vi "Play System Sound.vi"(8 "Error In":errorcluster, 11 "Windows Sound":T1) -> (0 "Error Out":errorcluster)   [LabVIEW 2021, in "Sound.lvlib"]
uses:
  Sound.lvlib
  System Sounds List.ctl
  <vilib>/Utility/sysdir.llb/System Directory Type.ctl
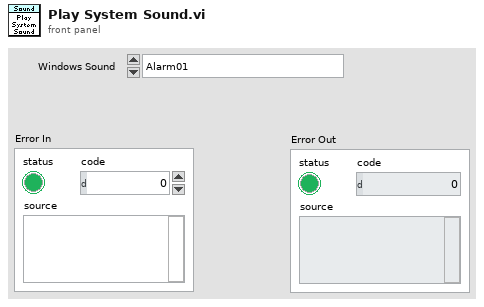
[diagram p1: front panel]
types:
  T1 = typedef "Sound.lvlib/System Sounds List.ctl" = enum16{"Alarm01", "Alarm02", "Alarm03", "Alarm04", "Alarm05", "Alarm06", "Alarm07", "Alarm08", "Alarm09", "Alarm10", "chimes", "chord", "ding", "notify", "recycle", "Ring01", "Ring02", "Ring03", "Ring04", "Ring05", "Ring06", "Ring07", "Ring08", "Ring09", "Ring10", "ringout", "Speech Off", "Speech On", "Speech Sleep", "tada", "Windows Background", "Windows Balloon", "Windows Battery Critical", "Windows Battery Low", "Windows Critical Stop", "Windows Default", "Windows Ding", "Windows Error", "Windows Exclamation", "Windows Feed Discovered", "Windows Foreground", "Windows Hardware Fail", "Windows Hardware Insert", "Windows Hardware Remove", "Windows Information Bar", "Windows Logoff Sound", "Windows Logon", "Windows Menu Command", "Windows Message Nudge", "Windows Minimize", "Windows Navigation Start", "Windows Notify Calendar", "Windows Notify Email", "Windows Notify Messaging", "Windows Notify System Generic", "Windows Notify", "Windows Pop-up Blocked", "Windows Print complete", "Windows Proximity Connection", "Windows Proximity Notification", "Windows Recycle", "Windows Restore", "Windows Ringin", "Windows Ringout", "Windows Shutdown", "Windows Startup", "Windows Unlock", "Windows User Account Control"}
  T2 = typedef "System Directory Type.ctl" = i32
  T3 = typedef "Sound Output Task ID.ctl" = u32
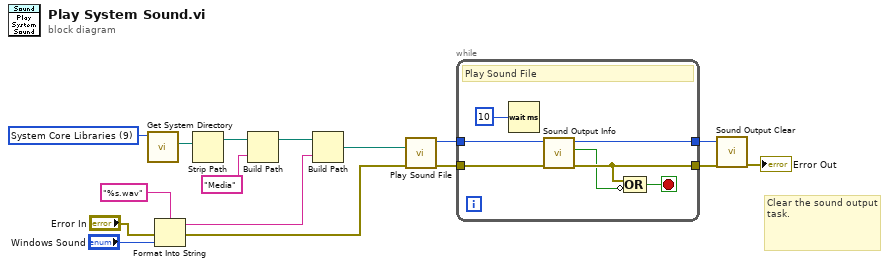
[diagram p0: block diagram]
diagram:
  w14 = T2 9 items=["User Home"=0, "User Desktop"=1, "User Documents"=2, "User Application Data"=3, "User Preferences"=4, "User Temporary"=5, "Public Documents"=6, "Public Application Data"=7, "Public Preferences"=8, "Public Cache"=13, "System Core Libraries"=9, "System Installed Libraries"=10, "Application Files"=11, "Boot Volume Root"=12] ("system directory type")
  # "Clear the sound output task."
  n1 = call <vilib>:"Get System Directory.vi"("system directory type"=w14) -> ("system directory"=w13:path)  [unwired: 10 in]
  n2 = Format Into String(format string="%s.wav", error in="Error In", "Windows Sound") -> (resulting string=w11:string, error out=w3:errorcluster)  [unwired: 1 in]
  n3 = Strip Path(path=w13) -> (stripped path=w12:path)  [unwired: 1 out]
  n4 = Build Path(base path=w12, name or relative path="Media") -> (appended path=w9:path)
  n5 = Build Path(base path=w9, name or relative path=w11) -> (appended path=w2:path)
  n6 = call <vilib>:"Play Sound File.vi"("error in (no error)"=w3, "path"=w2) -> ("error out"=w6:errorcluster, "task ID"=w7:T3)  [unwired: 8 in]
  n7 = while {
    tunnel: w7 -> [w18]
    tunnel: [w22] -> w4
    tunnel: w6 -> [w19]
    tunnel: [w21] -> w5
    stop <- w23 stop-if-true
    # "Play Sound File"
    n8 = Wait (ms)(milliseconds to wait=u32 10) -> ()  [unwired: 1 out]
    n9 = call <vilib>:"Sound Output Info.vi"("error in (no error)"=w19, "task ID"=w18) -> ("error out"=w21:errorcluster, "is playing?"=w20:bool, "task ID out"=w22:T3)  [unwired: 6 in, 1 out]
    n10 = Compound Arithmetic op=OR(w21, invert w20) -> (w23:bool)
  }
  n11 = call <vilib>:"Sound Output Clear.vi"("error in (no error)"=w5, "task ID"=w4) -> ("error out"=→"Error Out":errorcluster)  [unwired: 9 in]
